vi "Test VIignore.vi"() -> (0 "error out":errorcluster)   [LabVIEW 2020, in "UT_CICD.lvlib"]
uses:
  UT_CICD.lvlib
  Source/CICD.lvlib
panel:
  out "Filtered filenames":string[](array[string])
  out "number of files filtered":i32
  out "Filtered files":i32
  out "All files":i32
  out "VI paths filtered":path[](array[path])
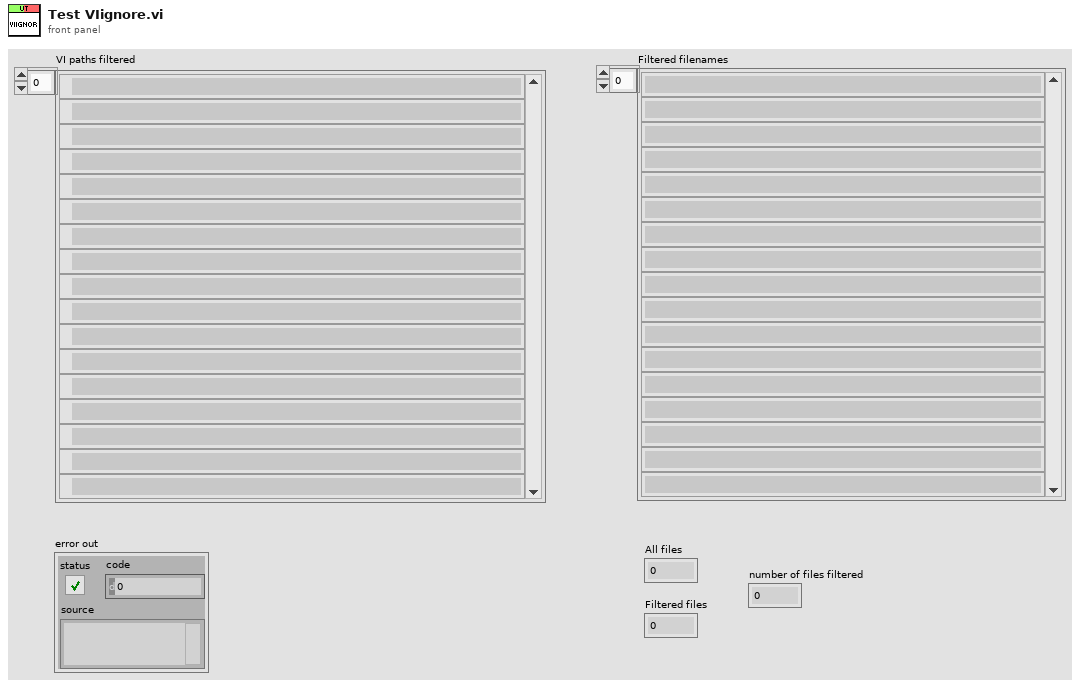
[diagram p1: front panel]
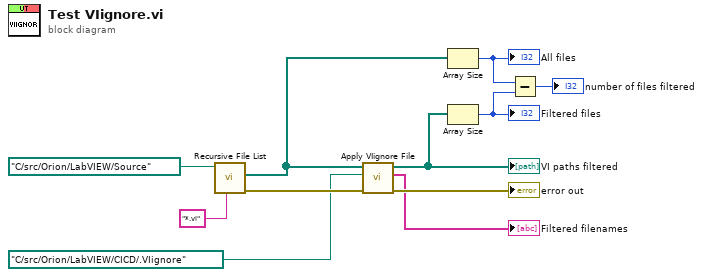
[diagram p0: block diagram]
diagram:
  n1 = call <vilib>:"Recursive File List.vi"("pattern"="*.vi", "Folder Path"=path "C:/src/Orion/LabVIEW/Source") -> ("error out"=w11:errorcluster, "All Files in Dir"=w6:path[])  [unwired: 5 in, 3 out]
  n2 = call "Apply VIignore File.vi"("error in"=w11, ".VIignore file"=path "C:/src/Orion/LabVIEW/CICD/.VIignore", "VI paths in"=w6) -> ("error out"=→"error out":errorcluster, "Filtered files"=→"Filtered filenames":string[], "VI paths filtered"=w5:path[])  [unwired: 6 in]
  "VI paths filtered" <- w5
  n3 = Array Size(array=w6) -> (size(s)=w4:i32)
  "All files" <- w4
  n4 = Array Size(array=w5) -> (size(s)=w3:i32)
  "Filtered files" <- w3
  n5 = Subtract(x=w4, y=w3) -> (x-y=→"number of files filtered":i32)
